vi "Set DOF Limits.vi"(4 "Limits  4":cluster{"Lower":dbl, "Upper":dbl, "Actual":dbl}, 5 "Limits 6":cluster{"Lower":dbl, "Upper":dbl, "Actual":dbl}, 6 "Limits 3":cluster{"Lower":dbl, "Upper":dbl, "Actual":dbl}, 7 "Limits 5":cluster{"Lower":dbl, "Upper":dbl, "Actual":dbl}, 8 "Limits 2":cluster{"Lower":dbl, "Upper":dbl, "Actual":dbl}, 9 "Limits 1":cluster{"Lower":dbl, "Upper":dbl, "Actual":dbl}, 10 "ID":T2, 11 "DofType":T1) -> ()   [LabVIEW 2013]
uses:
  Data Access Objects/Metadata/LBCB Number.ctl
  Data Access Objects/Limits/DofTypes.ctl
  Data Access Objects/Metadata/Cartesian Matrix.ctl
  Data Access Objects/Metadata/Cartesian Point.ctl
  Data Access Objects/Metadata/Actuator Matrix.ctl
  Data Access Objects/Metadata/Actuator Point.ctl
  Data Access Objects/Metadata/Persistant DAO Actions.ctl
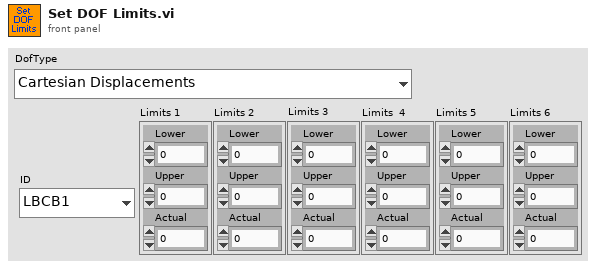
[diagram p1: front panel]
types:
  T1 = typedef "DofTypes.ctl" = enum16{"Cartesian Displacements", "Cartesian Forces & Moments", "Actuator Displacements", "Actuator Forces", "Cartesian Increments", "Actuator Increments"}
  T2 = typedef "LBCB Number.ctl" = enum16{"LBCB1", "LBCB2"}
  T3 = typedef "Cartesian Point.ctl" = cluster{"Dx":dbl, "Dy":dbl, "Dz":dbl, "Rx":dbl, "Ry":dbl, "Rz":dbl}
  T4 = typedef "Actuator Point.ctl" = cluster{"X1":dbl, "X2":dbl, "Y1":dbl, "Z1":dbl, "Z2":dbl, "Z3":dbl}
  T5 = typedef "Actuator Matrix.ctl" = cluster{"Lower":T4, "Upper":T4}
  T6 = typedef "Cartesian Matrix.ctl" = cluster{"Lower":T3, "Upper":T3}
  T7 = typedef "Persistant DAO Actions.ctl" = enum16{"Init", "Get", "Set", "Load", "Save"}
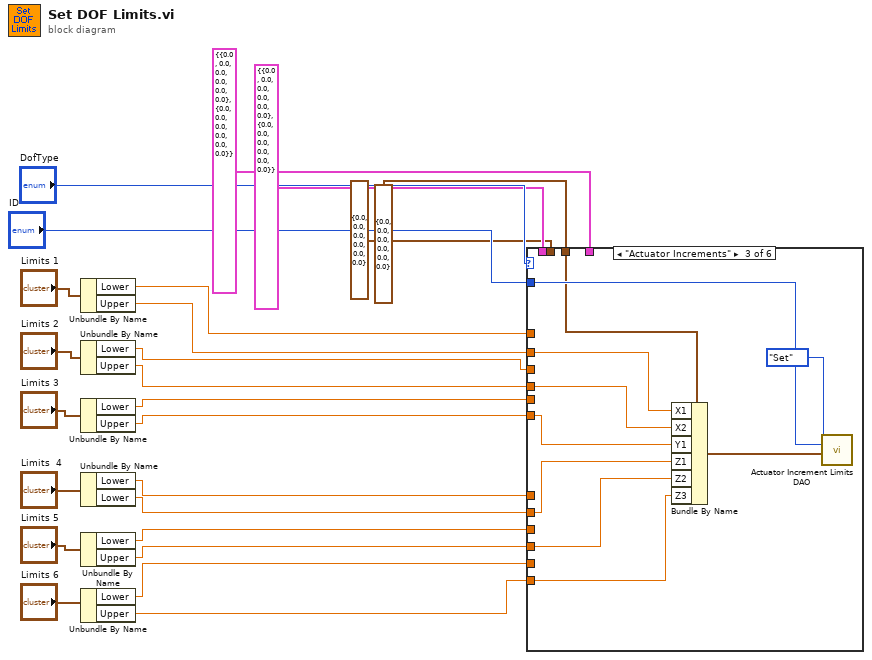
[diagram p0: block diagram]
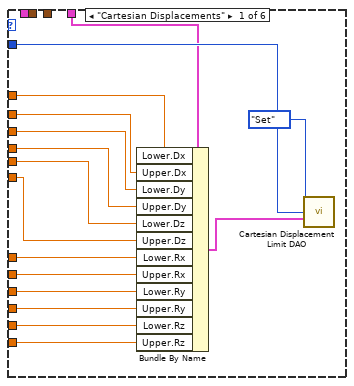
[diagram p2: hidden frame]
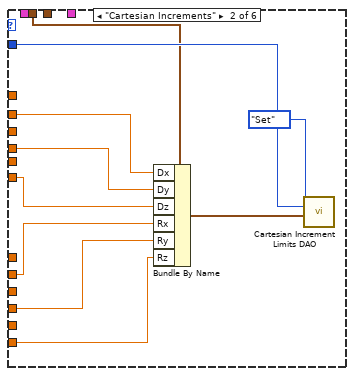
[diagram p3: hidden frame]
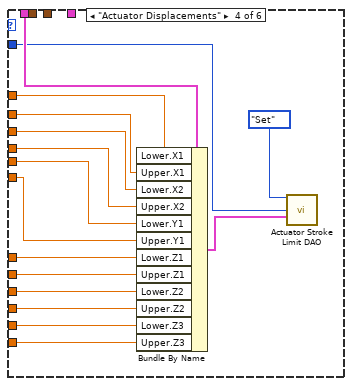
[diagram p4: hidden frame]
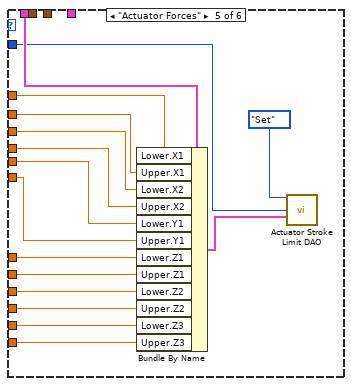
[diagram p5: hidden frame]
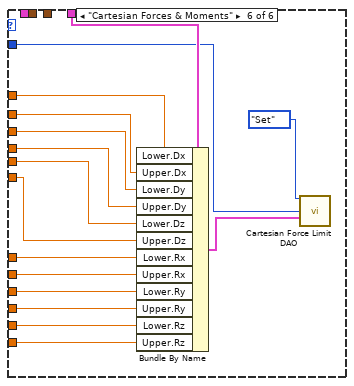
[diagram p6: hidden frame]
diagram:
  n1 = Unbundle By Name("Limits 1") -> ("Lower"=w15:dbl, "Upper"=w14:dbl)
  n2 = Unbundle By Name("Limits 2") -> ("Lower"=w13:dbl, "Upper"=w12:dbl)
  n3 = Unbundle By Name("Limits 3") -> ("Lower"=w11:dbl, "Upper"=w10:dbl)
  n4 = Unbundle By Name("Limits  4") -> ("Lower"=w9:dbl, "Lower"=w8:dbl)
  n5 = Unbundle By Name("Limits 5") -> ("Lower"=w7:dbl, "Upper"=w6:dbl)
  n6 = Unbundle By Name("Limits 6") -> ("Lower"=w5:dbl, "Upper"=w4:dbl)
  n7 = case shown="\"Actuator Increments\"" "DofType" {
    tunnel: "ID" -> [w39 w49 w59 w61 w77 w94]
    tunnel: T6 {"Lower"={"Dx"=0.0, "Dy"=0.0, "Dz"=0.0, "Rx"=0.0, "Ry"=0.0, "Rz"=0.0}, "Upper"={"Dx"=0.0, "Dy"=0.0, "Dz"=0.0, "Rx"=0.0, "Ry"=0.0, "Rz"=0.0}} ("Cartesian Displacement Out") -> [w38 _ _ _ _ w108]
    tunnel: w15 -> [w36 _ _ w76 w92 w107]
    tunnel: w14 -> [w35 w48 w58 w75 w91 w106]
    tunnel: w13 -> [w34 _ _ w74 w90 w105]
    tunnel: w12 -> [w33 w47 w57 w73 w89 w104]
    tunnel: w11 -> [w32 _ _ w72 w88 w103]
    tunnel: w10 -> [w31 w46 w56 w71 w87 w102]
    tunnel: w9 -> [w30 _ _ w70 w86 w101]
    tunnel: w8 -> [w29 w45 w55 w69 w85 w100]
    tunnel: w7 -> [w28 _ _ w68 w84 w99]
    tunnel: w6 -> [w27 w44 w54 w67 w83 w98]
    tunnel: w5 -> [w26 _ _ w66 w82 w97]
    tunnel: w4 -> [w25 w43 w53 w65 w81 w96]
    tunnel: T5 {"Lower"={"X1"=0.0, "X2"=0.0, "Y1"=0.0, "Z1"=0.0, "Z2"=0.0, "Z3"=0.0}, "Upper"={"X1"=0.0, "X2"=0.0, "Y1"=0.0, "Z1"=0.0, "Z2"=0.0, "Z3"=0.0}} ("Actuator Stroke Limits In") -> [_ _ _ w64 w80 _]
    tunnel: T4 {"X1"=0.0, "X2"=0.0, "Y1"=0.0, "Z1"=0.0, "Z2"=0.0, "Z3"=0.0} ("Upper") -> [_ _ w51 _ _ _]
    tunnel: T3 {"Dx"=0.0, "Dy"=0.0, "Dz"=0.0, "Rx"=0.0, "Ry"=0.0, "Rz"=0.0} ("Upper") -> [_ w42 _ _ _ _]
    frame "Cartesian Displacements" {
      n8 = Bundle By Name(cluster=w38, "Lower.Dx"=w36, "Upper.Dx"=w35, "Lower.Dy"=w34, "Upper.Dy"=w33, "Lower.Dz"=w32, "Upper.Dz"=w31, "Lower.Rx"=w30, "Upper.Rx"=w29, "Lower.Ry"=w28, "Upper.Ry"=w27, "Lower.Rz"=w26, "Upper.Rz"=w25) -> (w37:T6)
      n9 = call "Cartesian Displacement Limit DAO.vi"("Cartesian Displacement Limit Actions"=Persistant_DAO_Actions."Set", "ID"=w39, "Cartesian Displacement In"=w37) -> ()  [unwired: 10 in, 3 out]
    }
    frame "Cartesian Increments" {
      n10 = Bundle By Name(cluster=w42, "Dx"=w48, "Dy"=w47, "Dz"=w46, "Rx"=w45, "Ry"=w44, "Rz"=w43) -> (w41:T3)
      n11 = call "Cartesian Increment Limits DAO.vi"("Actions"=Persistant_DAO_Actions."Set" ("Cartesian Displacement Limit Actions"), "LBCB Number"=w49, "Inc Limits In"=w41) -> ()  [unwired: 10 in, 3 out]
    }
    frame "Actuator Increments" {
      n12 = Bundle By Name(cluster=w51, "X1"=w58, "X2"=w57, "Y1"=w56, "Z1"=w55, "Z2"=w54, "Z3"=w53) -> (w52:T4)
      n13 = call "Actuator Increment Limits DAO.vi"("Actions"=Persistant_DAO_Actions."Set" ("Cartesian Displacement Limit Actions"), "LBCB Number"=w59, "Inc Limits In"=w52) -> ()  [unwired: 10 in, 3 out]
    }
    frame "Actuator Displacements" {
      n14 = Bundle By Name(cluster=w64, "Lower.X1"=w76, "Upper.X1"=w75, "Lower.X2"=w74, "Upper.X2"=w73, "Lower.Y1"=w72, "Upper.Y1"=w71, "Lower.Z1"=w70, "Upper.Z1"=w69, "Lower.Z2"=w68, "Upper.Z2"=w67, "Lower.Z3"=w66, "Upper.Z3"=w65) -> (w62:T5)
      n15 = call "Actuator Stroke Limit DAO.vi"("Actuator Stroke Limit Actions"=Persistant_DAO_Actions."Set" ("Cartesian Displacement Limit Actions"), "ID"=w61, "Actuator Stroke Limits In"=w62) -> ()  [unwired: 10 in, 3 out]
    }
    frame "Actuator Forces" {
      n16 = Bundle By Name(cluster=w80, "Lower.X1"=w92, "Upper.X1"=w91, "Lower.X2"=w90, "Upper.X2"=w89, "Lower.Y1"=w88, "Upper.Y1"=w87, "Lower.Z1"=w86, "Upper.Z1"=w85, "Lower.Z2"=w84, "Upper.Z2"=w83, "Lower.Z3"=w82, "Upper.Z3"=w81) -> (w78:T5)
      n17 = call "Actuator Stroke Limit DAO.vi"("Actuator Stroke Limit Actions"=Persistant_DAO_Actions."Set" ("Cartesian Displacement Limit Actions"), "ID"=w77, "Actuator Stroke Limits In"=w78) -> ()  [unwired: 10 in, 3 out]
    }
    frame "Cartesian Forces & Moments" {
      n18 = Bundle By Name(cluster=w108, "Lower.Dx"=w107, "Upper.Dx"=w106, "Lower.Dy"=w105, "Upper.Dy"=w104, "Lower.Dz"=w103, "Upper.Dz"=w102, "Lower.Rx"=w101, "Upper.Rx"=w100, "Lower.Ry"=w99, "Upper.Ry"=w98, "Lower.Rz"=w97, "Upper.Rz"=w96) -> (w93:T6)
      n19 = call "Cartesian Force Limit DAO.vi"("Cartesian Force Limit Actions"=Persistant_DAO_Actions."Set" ("Cartesian Displacement Limit Actions"), "ID"=w94, "Cartesian Force Limit In"=w93) -> ()  [unwired: 10 in, 3 out]
    }
  }
